vi "PB-01 Read.vi"(6 "PB-01 in":T1={"FIFO Indexes"={"Write"={"Clear Faults"=0, "ESTTL Setup"=[], "UEGO Control"={"UEGO1Enable"=-1, "UEGO2Enable"=-1, "UEGO1Range"=-1, "UEGO2Range"=-1, "FilterCutoff (Hz)"=-1}}, "Read"={"UEGO Sensor Results"={"UEGO1Lambda"=-1, "UEGO1Phi"=-1, "UEGO1AFRatio"=-1, "UEGO1Ip (mA)"=-1, "UEGO2Lambda"=-1, "UEGO2Phi"=-1, "UEGO2AFRatio"=-1, "UEGO2Ip (mA)"=-1}, "UEGO Temperature (C)"={"UEGO1Temp (C)"=-1, "UEGO2Temp (C)"=-1, "UEGO1Hot"=-1, "UEGO2Hot"=-1}, "UEGO Diagnostics"={"UEGO1SensorFault"=-1, "UEGO2SensorFault"=-1, "UEGO1HeaterFault"=-1, "UEGO2HeaterFault"=-1, "UEGOFuseStatus"=-1, "Battery (V)"=-1, "LSUType"=-1}}}, "Settings"={"VR-Hall Mode Select"=[enum."VR Adaptive Arm", enum."VR Adaptive Arm", enum."VR Adaptive Arm", enum."VR Adaptive Arm", enum."VR Adaptive Arm"], "VR-Hall Arming Threshold [V]"=[0.0, 0.0, 0.0, 0.0, 0.0], "ESTTL Command Enabled"=FALSE}} {"FIFO Indexes"."Read"."UEGO Diagnostics"."LSUType" format="%02.0f"; "FIFO Indexes"."Read"."UEGO Diagnostics"."UEGOFuseStatus" format="%02.0f"}, 7 "Device Outputs in":dbl[](array[numeric]), 9 "UEGO Diagnostics":T4={"UEGO1SensorFault"=63, "UEGO2SensorFault"=63, "UEGO1HeaterFault"=192, "UEGO2HeaterFault"=192, "UEGOFuseStatus"=0, "Battery (V)"=0.0, "LSUType"=0} {"LSUType" items=["LSU 4.9", "LSU 4.2"]; "UEGOFuseStatus" items=["FUSE OK", "FUSE BLOWN"]; "UEGO2SensorFault" items=["NO FAULT"=63, "SHORT TO GND OR BATT"=0]; "UEGO2HeaterFault" items=["SHORT TO GROUND"=0, "OPEN CIRCUIT"=64, "SHORT TO BATTERY"=128, "NO FAULT"=192]; "UEGO1SensorFault" items=["NO FAULT"=63, "SHORT TO GND OR BATT"=0]; "UEGO1HeaterFault" items=["SHORT TO GROUND"=0, "OPEN CIRCUIT"=64, "SHORT TO BATTERY"=128, "NO FAULT"=192]}, 10 "UEGO Temperature (C)":T5, 11 "UEGO Sensor Results":T6) -> (5 "Device Outputs out":dbl[](array[numeric]))   [LabVIEW 2015]
uses:
  DCM-NIVS-RT/PB-01.ctl
  DCM-NIVS-RT/ESTTL Setup Indexes.ctl
  <vilib>/Powertrain Controls/Device Drivers/VR-Hall/RevC/Real-Time/Support/Vr_Hall_mode_control_revc.ctl
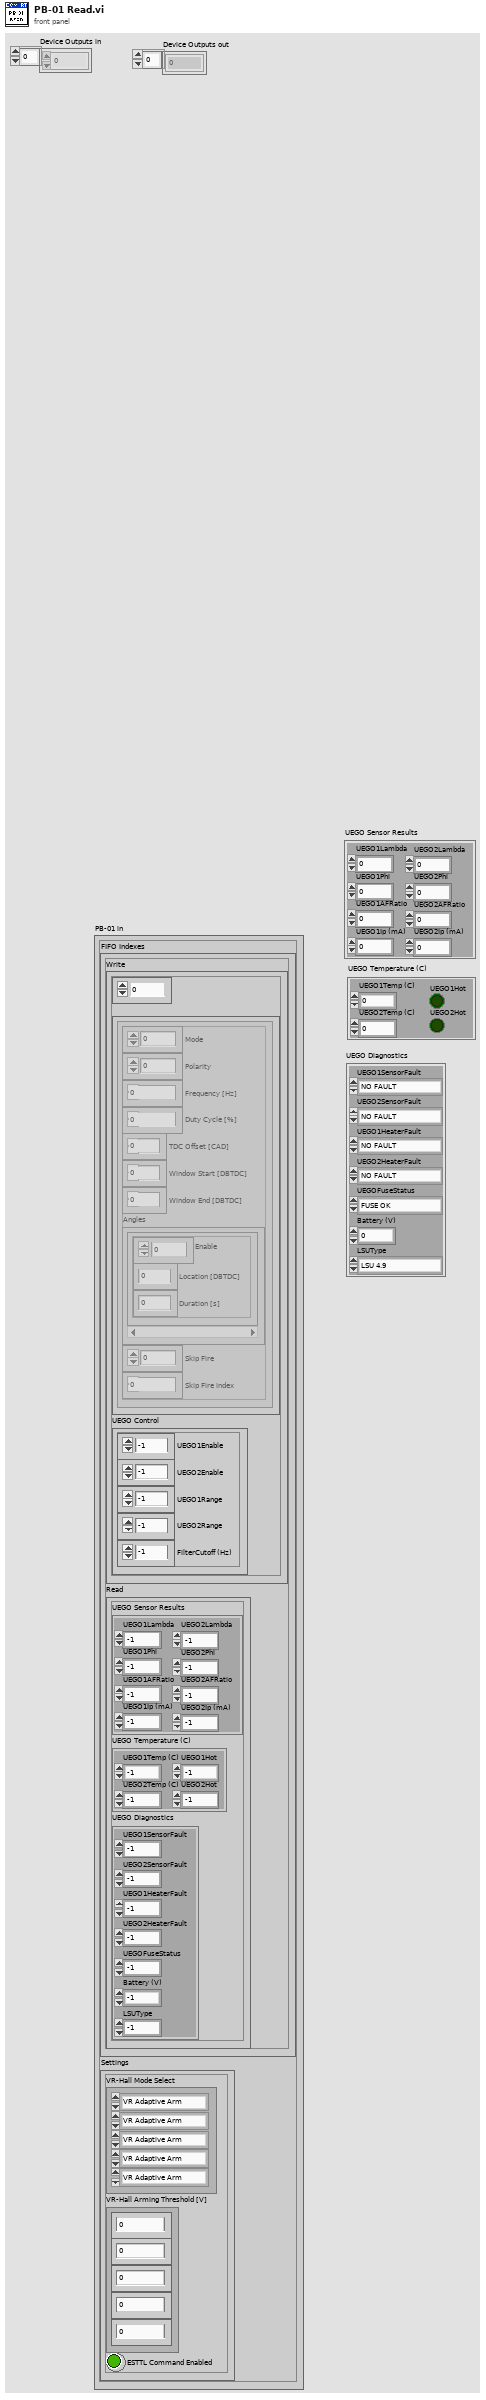
[diagram p1: front panel]
types:
  T1 = typedef "PB-01.ctl" = cluster{"FIFO Indexes":cluster{"Write":cluster{"Clear Faults":i32, "ESTTL Setup":T2[], "UEGO Control":cluster{"UEGO1Enable":i32, "UEGO2Enable":i32, "UEGO1Range":i32, "UEGO2Range":i32, "FilterCutoff (Hz)":i32}}, "Read":cluster{"UEGO Sensor Results":cluster{"UEGO1Lambda":i32, "UEGO1Phi":i32, "UEGO1AFRatio":i32, "UEGO1Ip (mA)":i32, "UEGO2Lambda":i32, "UEGO2Phi":i32, "UEGO2AFRatio":i32, "UEGO2Ip (mA)":i32}, "UEGO Temperature (C)":cluster{"UEGO1Temp (C)":i32, "UEGO2Temp (C)":i32, "UEGO1Hot":i32, "UEGO2Hot":i32}, "UEGO Diagnostics":cluster{"UEGO1SensorFault":i32, "UEGO2SensorFault":i32, "UEGO1HeaterFault":i32, "UEGO2HeaterFault":i32, "UEGOFuseStatus":i32, "Battery (V)":i32, "LSUType":i32}}}, "Settings":cluster{"VR-Hall Mode Select":T3[], "VR-Hall Arming Threshold [V]":dbl[], "ESTTL Command Enabled":bool}}
  T2 = typedef "ESTTL Setup Indexes.ctl" = cluster{"Mode":i32, "Polarity":i32, "Frequency [Hz]":i32, "Duty Cycle [%]":i32, "TDC Offset [CAD]":i32, "Window Start [DBTDC]":i32, "Window End [DBTDC]":i32, "Angles":cluster{"Enable":i32, "Location [DBTDC]":i32, "Duration [s]":i32}[], "Skip Fire":i32, "Skip Fire Index":i32}
  T3 = typedef "Vr_Hall_mode_control_revc.ctl" = enum32{"VR Adaptive Arm", "VR Manual Arm", "Hall", "Hall w/ Pull-up"}
  T4 = cluster{"UEGO1SensorFault":u8, "UEGO2SensorFault":u8, "UEGO1HeaterFault":u8, "UEGO2HeaterFault":u8, "UEGOFuseStatus":u8, "Battery (V)":sgl, "LSUType":u8}
  T5 = cluster{"UEGO1Temp (C)":sgl, "UEGO2Temp (C)":sgl, "UEGO1Hot":bool, "UEGO2Hot":bool}
  T6 = cluster{"UEGO1Lambda":sgl, "UEGO1Phi":sgl, "UEGO1AFRatio":sgl, "UEGO1Ip (mA)":sgl, "UEGO2Lambda":sgl, "UEGO2Phi":sgl, "UEGO2AFRatio":sgl, "UEGO2Ip (mA)":sgl}
  T7 = cluster{"UEGO1Lambda":i32, "UEGO1Phi":i32, "UEGO1AFRatio":i32, "UEGO1Ip (mA)":i32, "UEGO2Lambda":i32, "UEGO2Phi":i32, "UEGO2AFRatio":i32, "UEGO2Ip (mA)":i32}
  T8 = cluster{"UEGO1Temp (C)":i32, "UEGO2Temp (C)":i32, "UEGO1Hot":i32, "UEGO2Hot":i32}
  T9 = cluster{"UEGO1SensorFault":i32, "UEGO2SensorFault":i32, "UEGO1HeaterFault":i32, "UEGO2HeaterFault":i32, "UEGOFuseStatus":i32, "Battery (V)":i32, "LSUType":i32}
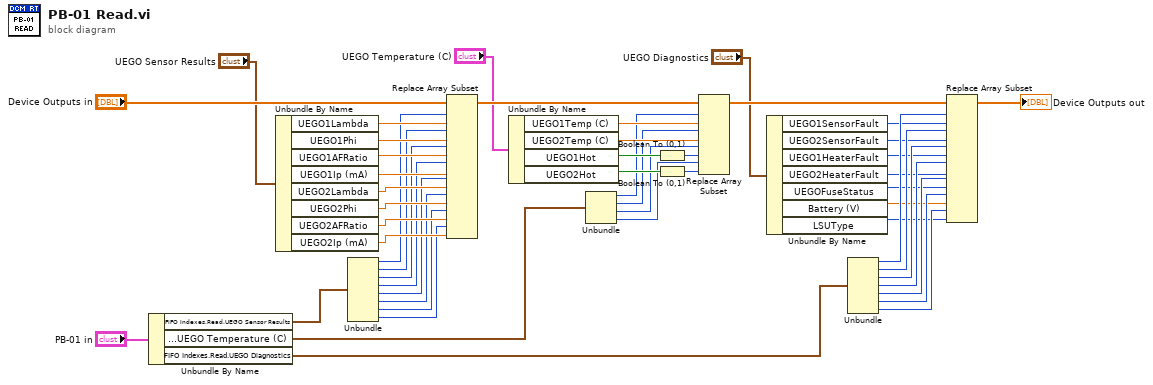
[diagram p0: block diagram]
diagram:
  n1 = Unbundle By Name("PB-01 in") -> ("FIFO Indexes.Read.UEGO Sensor Results"=w41:T7, "FIFO Indexes.Read.UEGO Temperature (C)"=w26:T8, "FIFO Indexes.Read.UEGO Diagnostics"=w3:T9)
  n2 = Unbundle By Name("UEGO Sensor Results") -> ("UEGO1Lambda"=w49:sgl, "UEGO1Phi"=w48:sgl, "UEGO1AFRatio"=w47:sgl, "UEGO1Ip (mA)"=w46:sgl, "UEGO2Lambda"=w45:sgl, "UEGO2Phi"=w44:sgl, "UEGO2AFRatio"=w43:sgl, "UEGO2Ip (mA)"=w42:sgl)
  n3 = Unbundle(w41) -> ("UEGO1Lambda"=w40:i32, "UEGO1Phi"=w39:i32, "UEGO1AFRatio"=w38:i32, "UEGO1Ip (mA)"=w37:i32, "UEGO2Lambda"=w36:i32, "UEGO2Phi"=w35:i32, "UEGO2AFRatio"=w34:i32, "UEGO2Ip (mA)"=w33:i32)
  n4 = Replace Array Subset(array="Device Outputs in", new element #1=w49, index #1=w40, new element #2=w48, index #2=w39, new element #3=w47, index #3=w38, new element #4=w46, index #4=w37, new element #5=w45, index #5=w36, new element #6=w44, index #6=w35, new element #7=w43, index #7=w34, new element #8=w42, index #8=w33) -> (w28:dbl[])
  n5 = Unbundle By Name("UEGO Temperature (C)") -> ("UEGO1Temp (C)"=w29:sgl, "UEGO2Temp (C)"=w30:sgl, "UEGO1Hot"=w31:bool, "UEGO2Hot"=w32:bool)
  n6 = Unbundle(w26) -> ("UEGO1Temp (C)"=w25:i32, "UEGO2Temp (C)"=w24:i32, "UEGO1Hot"=w22:i32, "UEGO2Hot"=w21:i32)
  n7 = Boolean To (0,1)(Boolean=w31) -> (0, 1=w23:i16)
  n8 = Boolean To (0,1)(Boolean=w32) -> (0, 1=w20:i16)
  n9 = Replace Array Subset(array=w28, new element #1=w29, index #1=w25, new element #2=w30, index #2=w24, new element #3=w23, index #3=w22, new element #4=w20, index #4=w21) -> (w5:dbl[])
  n10 = Unbundle By Name("UEGO Diagnostics") -> ("UEGO1SensorFault"=w6:u8, "UEGO2SensorFault"=w7:u8, "UEGO1HeaterFault"=w8:u8, "UEGO2HeaterFault"=w9:u8, "UEGOFuseStatus"=w10:u8, "Battery (V)"=w11:sgl, "LSUType"=w12:u8)
  n11 = Unbundle(w3) -> ("UEGO1SensorFault"=w13:i32, "UEGO2SensorFault"=w14:i32, "UEGO1HeaterFault"=w15:i32, "UEGO2HeaterFault"=w16:i32, "UEGOFuseStatus"=w17:i32, "Battery (V)"=w18:i32, "LSUType"=w19:i32)
  n12 = Replace Array Subset(array=w5, new element #1=w6, index #1=w13, new element #2=w7, index #2=w14, new element #3=w8, index #3=w15, new element #4=w9, index #4=w16, new element #5=w10, index #5=w17, new element #6=w11, index #6=w18, new element #7=w12, index #7=w19) -> (→"Device Outputs out":dbl[])
